vi "TEST - is OpenG.vi"(8 "error in (no error)":errorcluster) -> (0 "error out":errorcluster, 2 "pass":bool)   [LabVIEW 2009]
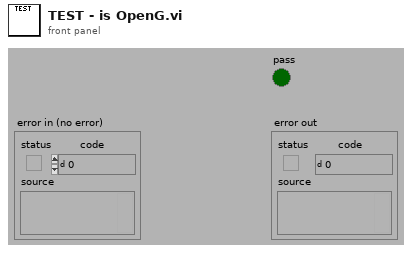
[diagram p1: front panel]
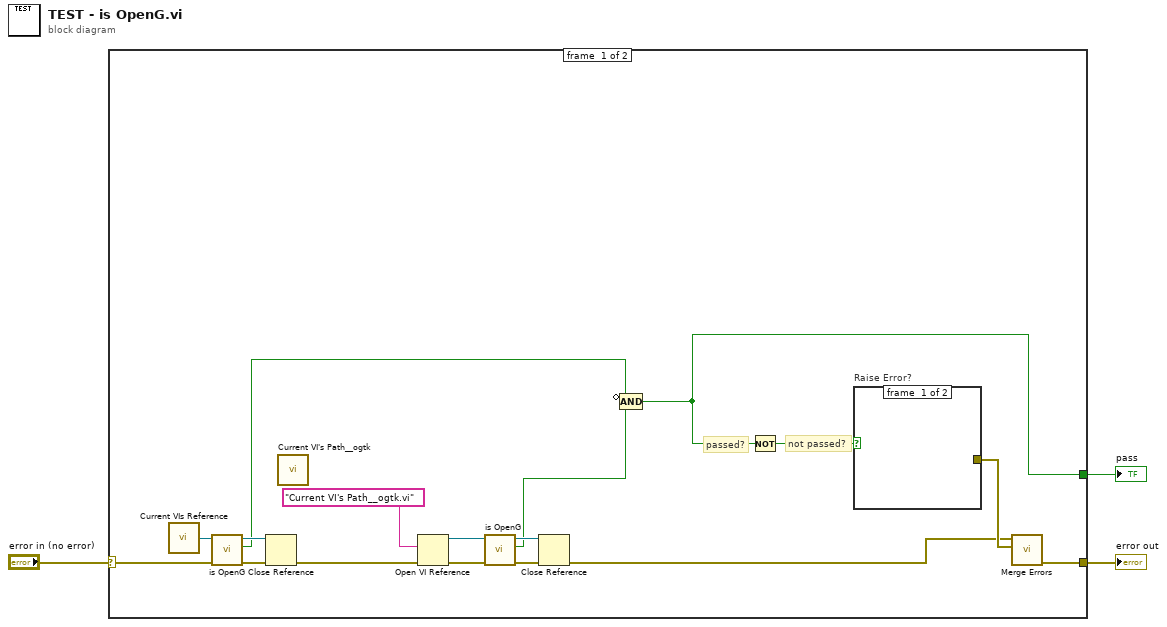
[diagram p0: block diagram]
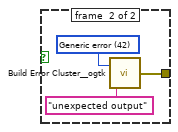
[diagram p2: hidden frame]
diagram:
  n1 = case shown="No Error" "error in (no error)" {
    selector: "error in (no error)" -> [w16 w24]
    tunnel: [w6 _] -> w3
    tunnel: [w20 w24] -> w1
    frame #0 {
      # "not passed?"
      # "passed?"
      n2 = call "Current VIs Reference.vi"() -> ("Current VI's reference"=w17:refnum<vi>)  [unwired: 5 in]
      n3 = call "is OpenG.vi"("error in (no error)"=w16, "VI reference"=w17) -> ("error out"=w15:errorcluster, "is OpenG VI?"=w8:bool, "dup VI reference"=w14:refnum<vi>)  [unwired: 7 in]
      n4 = Close Reference(reference=w14, error in (no error)=w15) -> (error out=w13:errorcluster)
      n5 = call <userlib>:"Current VI's Path__ogtk.vi"() -> ()  [unwired: 1 in, 1 out]
      n6 = Open VI Reference(vi path="Current VI's Path__ogtk.vi", error in (no error)=w13) -> (vi reference=w9:refnum<vi>, error out=w10:errorcluster)  [unwired: 4 in]
      n7 = call "is OpenG.vi"("error in (no error)"=w10, "VI reference"=w9) -> ("error out"=w11:errorcluster, "is OpenG VI?"=w7:bool, "dup VI reference"=w12:refnum<vi>)  [unwired: 7 in]
      n8 = Close Reference(reference=w12, error in (no error)=w11) -> (error out=w5:errorcluster)
      n9 = Compound Arithmetic op=AND(invert w8, w7) -> (w6:bool)
      n10 = Not(x=w6) -> (.not. x?=w18:bool)
      n11 = case "Raise Error?" shown="True" w18 {
        tunnel: [_ w21] -> w19
        frame #0 {
        }
        frame #1 {
          w22 = 42 items=["No error", "Argument error", "Memory is full", "Out of zone", "End of file", "File already open", "Generic file I/O error", "File not found", "File permission error", "Disk is full", "Duplicate path", "Too many files open", "System feature not enabled", "Resource file not found", "Cannot add resource", "Resource not found", "Image not found", "Image memory error", "Pen does not exist", "Config type invalid", "Config token not found", "Config parse error", "Config memory error", "Bad external code format", "Bad external code offset", "External code not present", "Null window", "Destroy window error", "Null menu", "Print aborted", "Bad print record", "Print driver error", "Windows error during printing", "Memory error during printing", "Print dialog error", "Generic print error", "Invalid device refnum", "Device not found", "Device parameter error", "Device unit error", "Cannot open device", "Device call aborted", "Generic error", "Cancelled by user", "Object ID too low", "Object ID too high", "Object not in heap", "Unknown heap", "Unknown object (invalid DefProc)", "Unknown object (DefProc not in table)", "Message out of range", "Invalid (null) method", "Unknown message", "Manager call not supported", "Bad address", "Network operation in progress", "Network operation timed out", "Connection is busy", "Network attribute not supported", "Network error", "Address in use", "System out of memory", "Connection aborted", "Connection refused", "Not connected", "Already connected", "Connection closed", "Initialization error (interapplication manager)", "Bad occurrence", "Wait on unbound occurrence handler", "Occurrence queue overflow", "Datalog type conflict", "Unused", "Unrecognized type (interapplication manager)", "Memory corrupt", "Failed to make temporary DLL", "Old CIN version", "Drag socket not found", "Failed to load drop-object", "Failed to register OLE object", "Failed to release OLE object", "Format specifier type mismatch", "Unknown format specifier", "Too few format specifiers", "Too many format specifiers", "Scan failed", "Newer CIN version", "Error converting to variant", "Runtime menu error", "Password tampered", "Variant attribute not found", "Incompatible variant data type", "Event data is not available", "Event Store is not present", "Occurrence is not found", "Event Queue is not created", "Event info is not available", "Refnum passed is NULL", "Error retrieving Class GUID", "Error retrieving CoClass GUID", "Error retrieving TypeLib GUID.", "Bad built application magic bytes.", "Specific driver is different from the specific driver associated with the Logical Name.", "There is no session opened to the class driver.", "Max Error", "MAX - Error with config objects", "MAX - Error loading configuration", "MAX - Group not supported"]
          n12 = call <userlib>:"Build Error Cluster__ogtk.vi"("String to Prepend to source (\"\")"="unexpected output" ("String to Prepend to source (\"\")"), "code"=w22) -> ("error out"=w21:errorcluster)
        }
      }
      n13 = call <vilib>:"Merge Errors.vi"("error in 2 (no error)"=w19, "error in 1 (no error)"=w5) -> ("error out"=w20:errorcluster)  [unwired: 5 in]
    }
    frame #1 {
    }
  }
  "pass" <- w3
  "error out" <- w1
